vi "XY Graph Sliced Mean, SDV & CV Enter Data Dialog.vi"(7 "Input Message":string, 8 "Error In":errorcluster, 10 "X min":dbl, 11 "X max":dbl) -> (0 "Error Out":errorcluster, 1 "Cancelled?":bool, 3 "Slices Definition":T1={"Axis Start"=0.0, "Axis Stop"=0.0, "# Steps"=0, "Step Size"=1.0, "Step Definition"=enum."# Steps", "Upper Percentile"=1.0, "Lower Percentile"=1.0, "Min # Data Points/Slice"=1, "Output Abscissa Statistics Plots"=FALSE, "Bin Location"=enum."Left"} {"Min # Data Points/Slice" min=0 max=100; "Lower Percentile" min=0.0 max=100.0; "Upper Percentile" min=0.0 max=100.0; "Step Size" min=1.0; "# Steps" min=1})   [LabVIEW 2021, in "XY Graph Add-Ons.lvlib"]
uses:
  XY Graph Add-Ons.lvlib
  XY Graph Sliced Mean & SDV Step Definition.ctl
  XY Graph Sliced CV Abscissa Location.ctl
panel:
  in  "Use Data Min/Max":bool
  in  "Slices Definition 2":T1={"Axis Start"=0.0, "Axis Stop"=0.0, "# Steps"=1, "Step Size"=1.0, "Step Definition"=enum."# Steps", "Upper Percentile"=100.0, "Lower Percentile"=0.0, "Min # Data Points/Slice"=1, "Output Abscissa Statistics Plots"=FALSE, "Bin Location"=enum."Left"} {"Min # Data Points/Slice" min=1; "Lower Percentile" min=0.0 max=100.0; "Upper Percentile" min=0.0 max=100.0; "Step Size" min=0.0; "# Steps" min=1}
  out "Message":string="Enter the first (start) and last (stop) values to consider for the analysis, as well as the number of intervals (# Steps) in which to divide the range of values:"
  in  "Cancel":bool
  in  "OK":bool
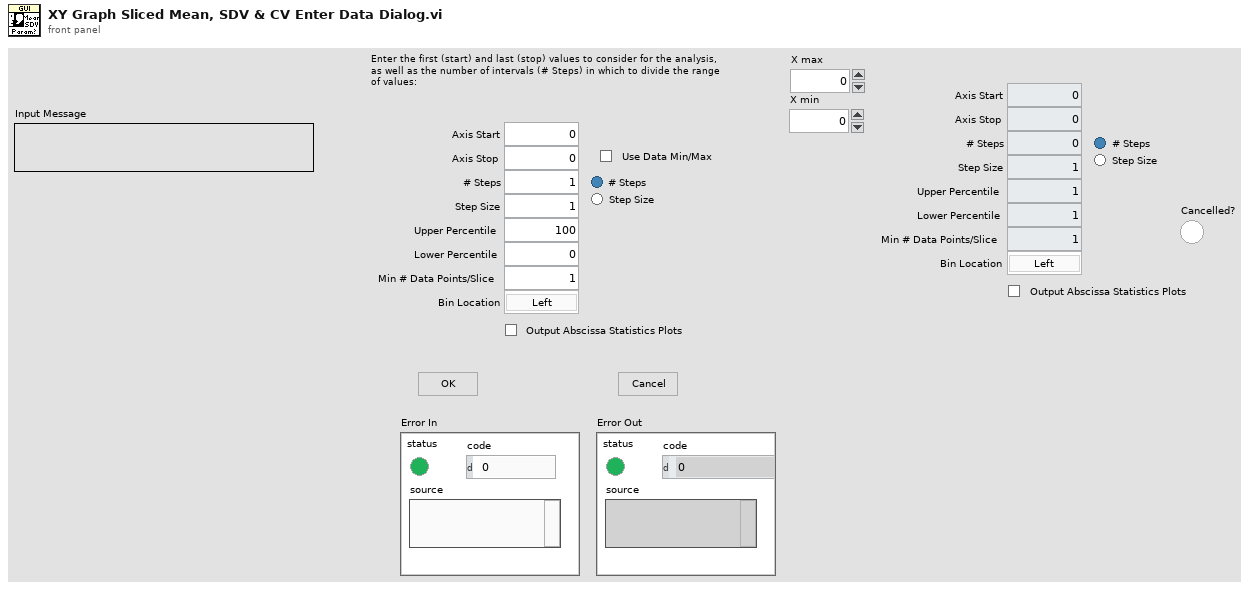
[diagram p1: front panel]
types:
  T1 = typedef "XY Graph Add-Ons.lvlib/XY Graph Sliced Mean & SDV Step Definition.ctl" = cluster{"Axis Start":dbl, "Axis Stop":dbl, "# Steps":i32, "Step Size":dbl, "Step Definition":enum32{"# Steps", "Step Size"}, "Upper Percentile":dbl, "Lower Percentile":dbl, "Min # Data Points/Slice":i32, "Output Abscissa Statistics Plots":bool, "Bin Location":T2}
  T2 = typedef "XY Graph Add-Ons.lvlib/XY Graph Sliced CV Abscissa Location.ctl" = enum16{"Left", "Center", "Mean", "Right"}
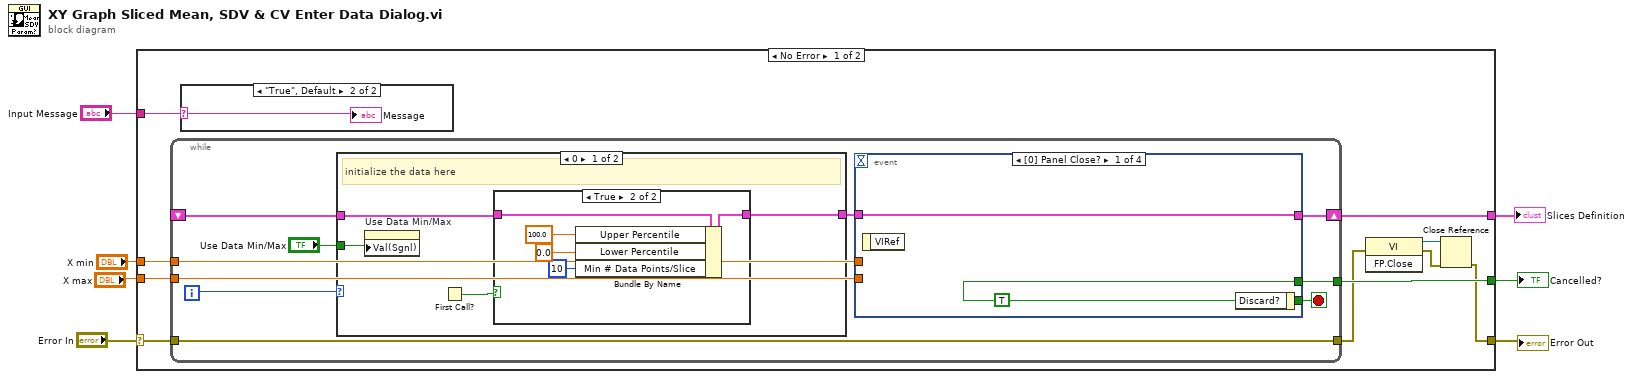
[diagram p0: block diagram]
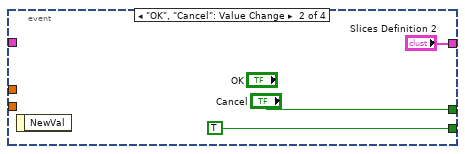
[diagram p5: hidden frame]
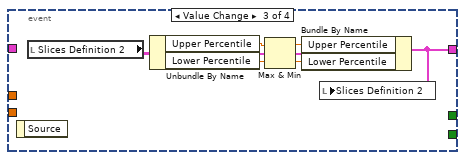
[diagram p6: hidden frame]
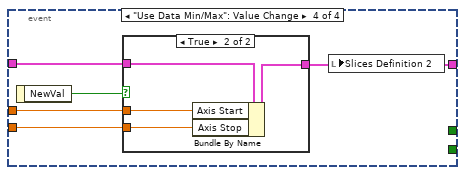
[diagram p7: hidden frame]
diagram:
  n1 = case shown="No Error" "Error In" {
    selector: "Error In" -> [w12 w61]
    tunnel: [w17 _] -> w7
    tunnel: [w16 _] -> w3
    tunnel: "Input Message" -> [w8 _]
    tunnel: [w13 w61] -> w4
    tunnel: "X min" -> [w10 _]
    tunnel: "X max" -> [w9 _]
    frame No Error {
      n2 = while {
        tunnel: [w27] -> w17
        shift-right: [w24] -> w16
        shift-left: _ -> [w25]
        tunnel: w12 -> [w22]
        tunnel: [w22] -> w11
        tunnel: w10 -> [w21]
        tunnel: w9 -> [w20]
        i -> [w26]
        stop <- w28 stop-if-true
        n3 = case shown="0" w26 {
          tunnel: w25 -> [w30 w39]
          tunnel: [w31 w39] -> w23
          tunnel: "Use Data Min/Max" -> [w29 _]
          frame 0 {
            # "initialize the data here"
            n4 = property on="Use Data Min/Max" class="Bool (strict)"("Val(Sgnl)"=w29) -> ()  [unwired: 2 in, 2 out]
            n5 = First Call?() -> (First Call?: T/F=w32:bool)
            n6 = case shown="True" w32 {
              tunnel: w30 -> [w33 w38]
              tunnel: [w33 w37] -> w31
              frame False {
              }
              frame True {
                n7 = Bundle By Name(cluster=w38, "Upper Percentile"=100.0, "Lower Percentile"=0.0, "Min # Data Points/Slice"=10) -> (w37:T1)
              }
            }
          }
          frame 1, Default {
          }
        }
        n8 = event shown="[0] Panel Close?" {
          selector: _ -> [_ _ _ _]
          dyn-events: _ -> [_ _ _ _]
          timeout: _ -> [_ _ _ _]
          tunnel: [w41 TRUE ("Discard?") _ _] -> w28
          tunnel: [w41 "Cancel" _ _] -> w27
          tunnel: [w40 "Slices Definition 2" w45 w52] -> w24
          tunnel: w23 -> [w40 _ _ w55]
          tunnel: w21 -> [_ _ _ w54]
          tunnel: w20 -> [_ _ _ w53]
          event Panel Close? {
            w41 = TRUE ("Discard?")
            n9 = event-data() -> ()  [unwired: 1 in, 1 out]
            n10 = event-data("Discard?"=w41) -> ()  [unwired: 1 in, 1 out]
          }
          event "OK", "Cancel": Value Change {
            n11 = event-data() -> ()  [unwired: 1 in, 1 out]
          }
          event Value Change {
            n12 = event-data() -> ()  [unwired: 1 in, 1 out]
            n13 = local read "Slices Definition 2"() -> (w48:T1)
            n14 = Unbundle By Name(w48) -> ("Upper Percentile"=w50:dbl, "Lower Percentile"=w49:dbl)
            n15 = Max & Min(x=w50, y=w49) -> (max(x,y)=w47:dbl, min(x,y)=w46:dbl)
            n16 = Bundle By Name(cluster=w48, "Upper Percentile"=w47, "Lower Percentile"=w46) -> (w45:T1)
            n17 = local write "Slices Definition 2"(w45) -> ()
          }
          event "Use Data Min/Max": Value Change {
            n18 = event-data() -> ("NewVal"=w51:bool)  [unwired: 1 in]
            n19 = case shown="True" w51 {
              tunnel: w55 -> [w56 w60]
              tunnel: w54 -> [_ w59]
              tunnel: w53 -> [_ w58]
              tunnel: [w56 w57] -> w52
              frame False {
              }
              frame True {
                n20 = Bundle By Name(cluster=w60, "Axis Start"=w59, "Axis Stop"=w58) -> (w57:T1)
              }
            }
            n21 = local write "Slices Definition 2"(w52) -> ()
          }
        }
      }
      n22 = case shown="\"True\", Default" w8 {
        selector: w8 -> [_ w18]
        frame "" {
        }
        frame "True", Default {
          "Message" <- w18
        }
      }
      n23 = invoke class="VI" method="FP.Close"(error in=w11) -> (reference out=w15:refnum<vi>, error out=w14:errorcluster)  [unwired: 2 in, 1 out]
      n24 = Close Reference(reference=w15, error in (no error)=w14) -> (error out=w13:errorcluster)
    }
    frame Error {
    }
  }
  "Cancelled?" <- w7
  "Error Out" <- w4
  "Slices Definition" <- w3
